vi "MainIteratesTempForResonance.vi"() -> ()   [LabVIEW 2010]
panel:
  in  "#Measurements each Frequency":i32=200
  out "error out":errorcluster
  in  "error in":errorcluster
  in  "Step":dbl=200.0 format="%.2f"
  in  "Start":dbl=200.0 format="%.2f"
  in  "Stop":dbl=200.0 format="%.2f"
  in  "Voltage Stop":dbl=200.0 format="%.2f"
  in  "Voltage Step":dbl=200.0 format="%.2f"
  in  "Voltage Start":dbl=200.0 format="%.2f"
  in  "Wait equilibrium (min)":dbl=200.0 format="%.2f"
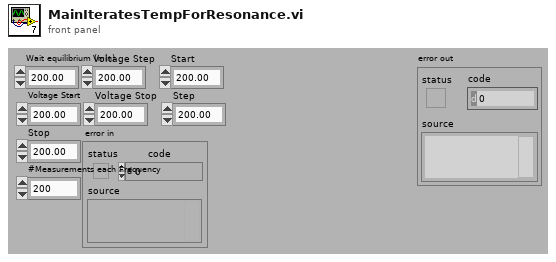
[diagram p1: front panel]
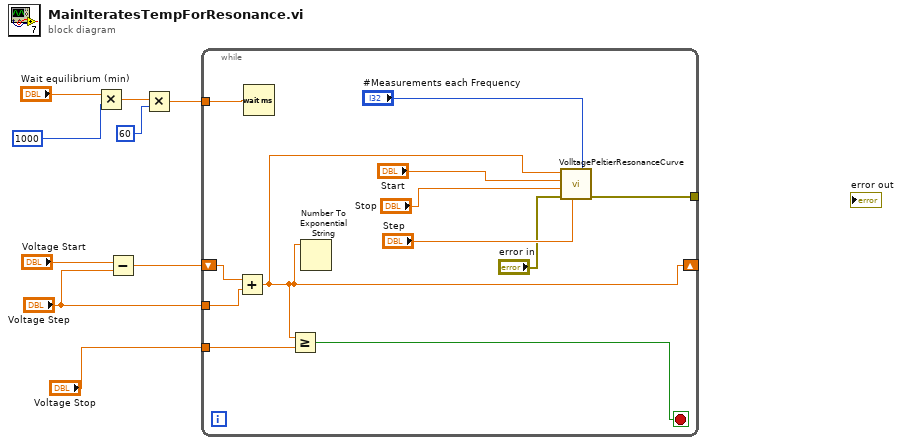
[diagram p0: block diagram]
diagram:
  n1 = Multiply(x="Wait equilibrium (min)", y=1000) -> (x*y=w7:dbl)
  n2 = Subtract(x="Voltage Start", y="Voltage Step") -> (x-y=w3:dbl)
  n3 = Multiply(x=w7, y=60) -> (x*y=w5:dbl)
  n4 = while {
    tunnel: w5 -> [w21]
    shift-right: [w11] -> _
    shift-left: w3 -> [w19]
    tunnel: "Voltage Step" -> [w20]
    tunnel: "Voltage Stop" -> [w18]
    tunnel: [w16] -> _
    stop <- w17 stop-if-true
    n5 = Add(x=w19, y=w20) -> (x+y=w11:dbl)
    n6 = Wait (ms)(milliseconds to wait=w21) -> ()  [unwired: 1 out]
    n7 = Greater Or Equal?(x=w11, y=w18) -> (x >= y?=w17:bool)
    n8 = Number To Exponential String(number=w11) -> ()  [unwired: 3 in, 1 out]
    n9 = call "VolltagePeltierResonanceCurve.vi"("#Measurements each Frequency"="#Measurements each Frequency", "Step"="Step", "error in"="error in", "Stop"="Stop", "Start"="Start", "Voltage"=w11) -> ("error out"=w16:errorcluster)  [unwired: 5 in]
  }
